vi "Get Response (SubVI).vi"(8 "error in (no error)":errorcluster, 10 "timeout ms (25000)":i32=10, 11 "TCP Network Connection in":refnum<k5>) -> (0 "error out":errorcluster, 2 "Response data":string="0223400010514;001;608/484;804/483;805/553;609/559;706/520,400010511;004;611/702;806/702;807/763;611/763;709/732,400010511;002;891/488;1087/493;1087/548;891/548;989/520,400010514;003;892/699;1088/698;1089/769;893/770;990/734", 3 "TCP Network Connection out":refnum<k5>)   [LabVIEW 2019, in "SR_2000.lvlib"]
uses:
  SR_2000.lvlib
panel:
  out "length":i32=223
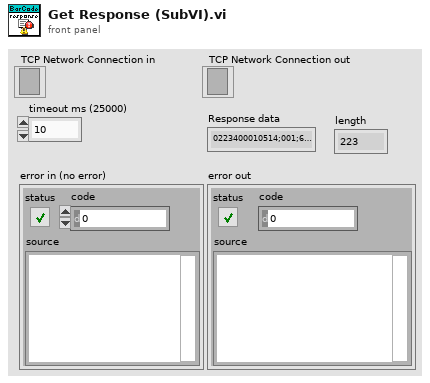
[diagram p1: front panel]
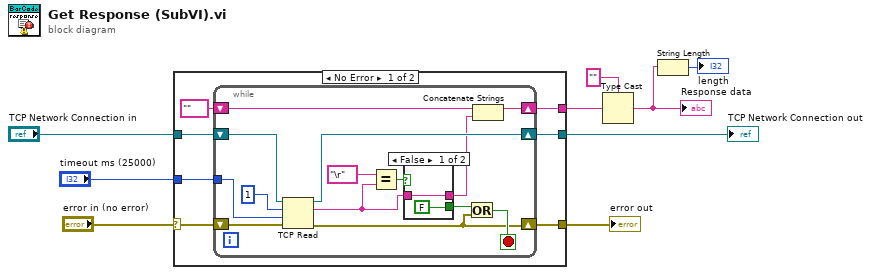
[diagram p0: block diagram]
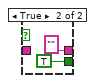
[diagram p2: hidden frame]
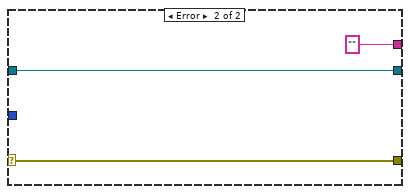
[diagram p3: hidden frame]
diagram:
  n1 = case shown="No Error" "error in (no error)" {
    selector: "error in (no error)" -> [w11 w37]
    tunnel: [w16 w37] -> w4
    tunnel: "TCP Network Connection in" -> [w15 w36]
    tunnel: [w13 ""] -> w8
    tunnel: [w12 w36] -> w6
    tunnel: "timeout ms (25000)" -> [w10 _]
    frame No Error {
      n2 = while {
        shift-right: [w18] -> w16
        shift-left: w11 -> [w30]
        shift-right: [w26] -> w13
        shift-left: "" -> [w27]
        shift-right: [w25] -> w12
        shift-left: w15 -> [w28]
        tunnel: w10 -> [w17]
        stop <- w19 stop-if-true
        n3 = TCP Read(connection ID=w28, bytes to read=1, error in (no error)=w30, 9:w17) -> (connection ID out=w25:refnum<k5>, data out=w21:string, error out=w18:errorcluster)  [unwired: 1 in]
        n4 = Equal?(x="\r" ("y"), y=w21) -> (x = y?=w24:bool)
        n5 = case shown="False" w24 {
          tunnel: [FALSE ("f") TRUE] -> w20
          tunnel: w21 -> [w31 _]
          tunnel: [w31 "" ("data out")] -> w22
          frame False {
          }
          frame True {
          }
        }
        n6 = Or(x=w20, y=w18) -> (x .or. y?=w19:bool)
        n7 = Concatenate Strings(w27, w22) -> (w26:string)
      }
    }
    frame Error {
    }
  }
  "TCP Network Connection out" <- w6
  "error out" <- w4
  n8 = Type Cast(type="", x=w8) -> (*(type *) &x=w3:string)
  "Response data" <- w3
  n9 = String Length(string=w3) -> (length=→"length":i32)
